vi "Insert View.vi"(8 "error in (no error)":errorcluster, 9 "Insertion Request Time":timestamp, 10 "Protected Subpanel":T1, 11 "MultiSubscriber In":refnum<class "MultiSubscriber.lvclass">) -> (0 "error out":errorcluster, 3 "MultiSubscriber Out":refnum<class "MultiSubscriber.lvclass">)   [LabVIEW 2015, in "TestViewables.lvlib" / "MultiSubscriber.lvclass"]
doc: "<License>\nCopyright © 2017 Composed Systems, LLC | All rights reserved\nwww.composed.io\n\nAuthor: Ethan Stern <ethan.stern@composed.io>\n\nThis software is provided \"AS IS\" WITHOUT WARRANTIES, either express or implied, AND IS FOR EDUCATIONAL PURPOSES ONLY.\n</License>"
uses:
  MultiSubscriber.lvclass
  <vilib>/Composed Systems/Protected Subpanel/Protected Subpanel Reference.ctl
  <vilib>/Composed Systems/Protected Subpanel/ProtectedSubpanel.lvclass
  MultiSubscriber.lvclass/MultiSubscriber.ctl
  Framework/IViewable/IViewable/IViewable.lvclass
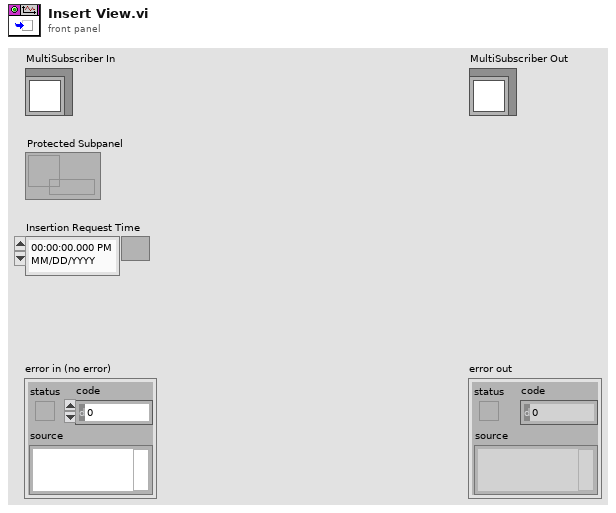
[diagram p1: front panel]
types:
  T1 = typedef "ProtectedSubpanel.lvlib/ProtectedSubpanel.lvclass/Protected Subpanel Reference.ctl" = refnum<data-value>
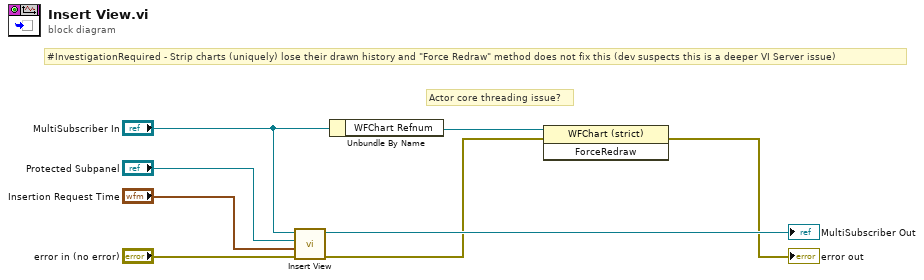
[diagram p0: block diagram]
diagram:
  # "Actor core threading issue?"
  # "#InvestigationRequired - Strip charts (uniquely) lose their drawn history and \"Force Redraw\" method does not fix this (dev suspects this is a deeper VI Server issue)"
  n1 = call-parent "Insert View.vi"("error in (no error)"="error in (no error)", "Insertion Request Time"="Insertion Request Time", "Protected Subpanel"="Protected Subpanel", "IViewable in"="MultiSubscriber In") -> ("error out"=w3:errorcluster, "IViewable out"=→"MultiSubscriber Out":refnum<class "MultiSubscriber.lvclass">)  [unwired: 6 in]
  n2 = Unbundle By Name("MultiSubscriber In") -> ("WFChart Refnum"=w4:refnum<vi>)
  n3 = invoke class="WFChart (strict)" method="ForceRedraw"(reference=w4, error in=w3) -> (error out=→"error out":errorcluster)  [unwired: 1 in, 2 out]
